vi "Multiplicate Matrix Size.vi"(10 "Times to multiply size":i32=4, 11 "Data Matrix In":u8[][](array[numeric])) -> (3 "Data Matrix Out":u8[][](array[numeric]))   [LabVIEW 2019, in "Day 15.lvlib"]
uses:
  Day 15.lvlib
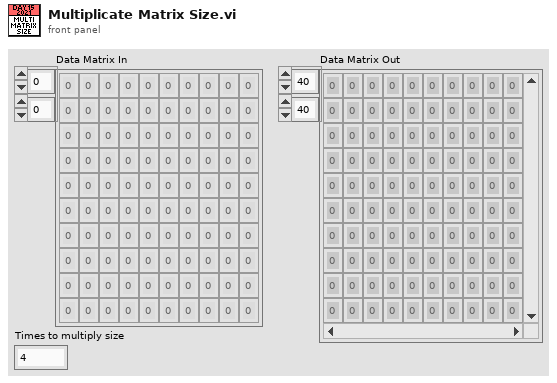
[diagram p1: front panel]
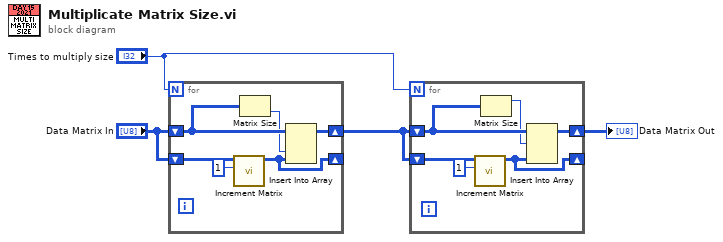
[diagram p0: block diagram]
diagram:
  n1 = for {
    N: "Times to multiply size" -> [_]
    shift-right: [w9] -> w2
    shift-left: "Data Matrix In" -> [w10]
    shift-right: [w6] -> _
    shift-left: "Data Matrix In" -> [w8]
    n2 = call "Increment Matrix.vi"("Value to add"=u8 1, "Data Matrix In"=w8) -> ("Data Matrix Out"=w6:u8[][])  [unwired: 9 in]
    n3 = Matrix Size(0:w10) -> (2:w7:i32)  [unwired: 1 out]
    n4 = Insert Into Array(array=w10, index (col)=w7, new element=w6) -> (w9:u8[][])  [unwired: 1 in]
  }
  n5 = for {
    N: "Times to multiply size" -> [_]
    shift-right: [w15] -> w1
    shift-left: w2 -> [w16]
    shift-right: [w12] -> _
    shift-left: w2 -> [w14]
    n6 = call "Increment Matrix.vi"("Value to add"=u8 1, "Data Matrix In"=w14) -> ("Data Matrix Out"=w12:u8[][])  [unwired: 9 in]
    n7 = Matrix Size(0:w16) -> (1:w13:i32)  [unwired: 1 out]
    n8 = Insert Into Array(array=w16, index (row)=w13, new element=w12) -> (w15:u8[][])  [unwired: 1 in]
  }
  "Data Matrix Out" <- w1
